vi "PCO_SetRecordingState.vi"(8 "error in (no error)":errorcluster, 10 "wRecState":enum16{"stop", "run"}(ring), 11 "Handle":u64) -> (0 "error out":errorcluster, 3 "Handle Out":u64, 5 "return type":u32 format="%x")   [LabVIEW 2011]
uses:
  SC2_Cam64.dll
panel:
  # "C0031002: already off"
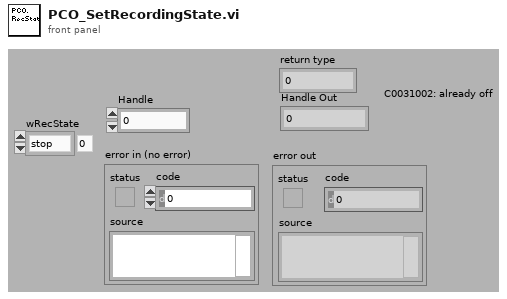
[diagram p1: front panel]
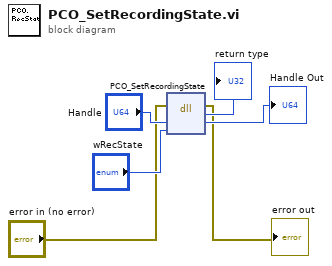
[diagram p0: block diagram]
diagram:
  n1 = dll-call lib="SC2_Cam*.*" fn="PCO_SetRecordingState"(error in="error in (no error)", "Handle"="Handle", "wRecState"="wRecState") -> (error out=→"error out":errorcluster, "return type"=→"return type":u32, "Handle"=→"Handle Out":u64)  [unwired: 2 in, 2 out]
